vi "Get DDGTTL Gate Width.vi"(10 "ttlWidth":cluster{}, 11 "opticalWidth":cluster{}) -> (2 "ttlWidth out":cluster{}, 3 "function return":u32)   [LabVIEW 2018, in "Copy of Andor SDK.lvlib"]
doc: "EXPNETTYPE unsigned int WINAPI GetDDGTTLGateWidth(at_u64 opticalWidth, at_u64 * ttlWidth);"
uses:
  Copy of Andor SDK.lvlib
  <userlib>/Andor SDK/ATMCD32D.dll
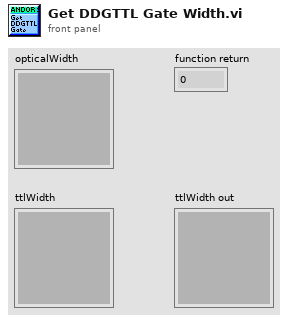
[diagram p1: front panel]
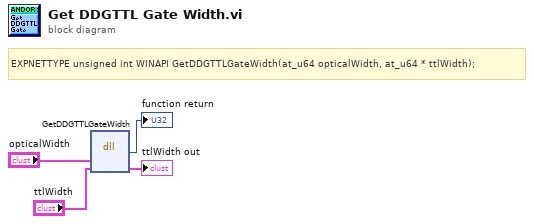
[diagram p0: block diagram]
diagram:
  # "EXPNETTYPE unsigned int WINAPI GetDDGTTLGateWidth(at_u64 opticalWidth, at_u64 * ttlWidth);"
  n1 = dll-call lib="C:/Program Files (x86)/National Instruments/LabVIEW 2018/user.lib/Andor SDK/ATMCD32D.*" fn="GetDDGTTLGateWidth"("opticalWidth"="opticalWidth", "ttlWidth"="ttlWidth") -> (→"function return":u32, "ttlWidth"=→"ttlWidth out":cluster{})  [unwired: 4 in, 2 out]
